vi "Configure Decimator 0.vi"(7 "lock-in.decimator0 0":i32, 8 "error in (no error)":errorcluster, 10 "lock-in.decimation0 0":i32, 11 "LIA Host Interface in":refnum<class "LIA Debugging.lvclass">) -> (0 "error out":errorcluster, 3 "LIA Host Interface out":refnum<class "LIA Debugging.lvclass">)   [LabVIEW 2017, in "LIA Debugging.lvclass"]
uses:
  LIA Debugging.lvclass
  Program Files (x86)/National Instruments/LabVIEW 2017/examples/Lock-In Amplifier/lib/interface/Interface FPGA/LIA Host Interface FPGA.lvclass
  Program Files (x86)/National Instruments/LabVIEW 2017/examples/Lock-In Amplifier/lib/interface/Interface FPGA/Properties/FpgaSession_GET.vi
  <vilib>/Utility/error.llb/Error Cluster From Error Code.vi
  <vilib>/rvi/errors/niLvFpgaAdjustHostInterfaceError.vi
  <vilib>/rvi/interface/nirviReadWriteControl/nirviReadWriteControl.xnode
  NiFpgaLv.dll
  <vilib>/rvi/interface/Simulation/niFpgaSimulationCallBeginRW.vi
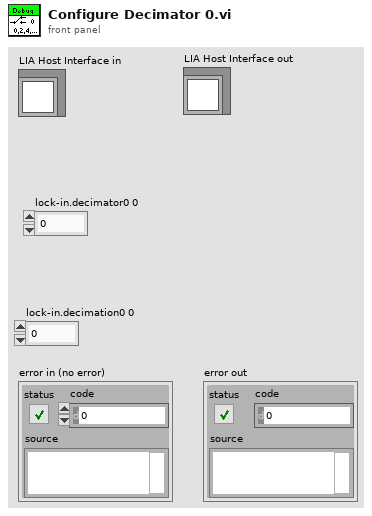
[diagram p1: front panel]
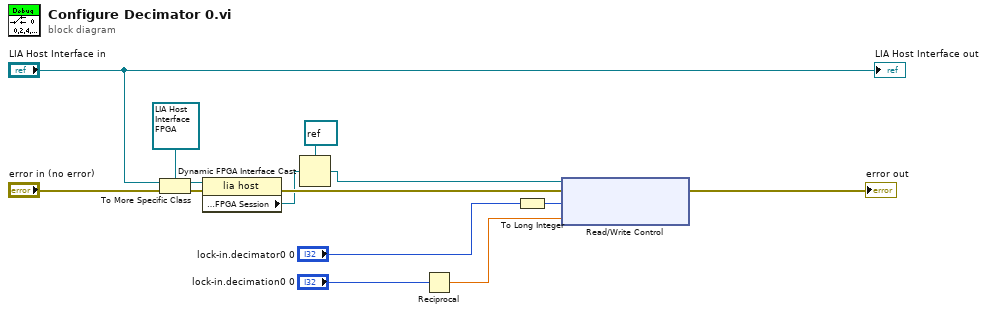
[diagram p0: block diagram]
diagram:
  n1 = To More Specific Class(target class=refnum<class "LIA Host Interface FPGA.lvclass"> refnum ("lia host"), reference="LIA Host Interface in", error in="error in (no error)") -> (specific class reference=w9:refnum<class "LIA Host Interface FPGA.lvclass">, error out=w8:errorcluster)
  n2 = property class="lia host"(reference=w9, error in=w8) -> (error out=w14:errorcluster, "Properties:FPGA Session"=w10:refnum<k20>)  [unwired: 1 out]
  n3 = Dynamic FPGA Interface Cast(Session In=refnum<k20> refnum ("fpga type"), Type=w10) -> (Session Out=w4:refnum<k20>)
  n4 = Reciprocal(x="lock-in.decimation0 0") -> (1/x=w13:dbl)
  n5 = To Long Integer(number="lock-in.decimator0 0") -> (32bit integer=w2:i32)
  n6 = xnode "Read/Write Control"("FPGA VI Reference In"=w4, "error in"=w14, "lock-in.decimator0 0"=w2, "lock-in.fir0 fs 0"=w13) -> ("error out"=→"error out":errorcluster)  [unwired: 1 out]
  "LIA Host Interface out" <- "LIA Host Interface in"
